vi "Update Tag String.vi"(8 "error in (no error)":errorcluster, 9 "string":string caption="String", 10 "Tag Path":string, 11 "Logger in.lvclass":refnum<class "Logger.lvclass">) -> (0 "error out":errorcluster, 3 "Logger out.lvclass":refnum<class "Logger.lvclass">)   [LabVIEW 2023, in "Logger.lvclass"]
uses:
  Logger.lvclass
  Logger.lvclass/Logger.ctl
  <vilib>/Skyline/Tag/Wrapper/Wrapper_class/Generate Tag Cluster (String) 2.vi
  <vilib>/Skyline/Tag/Wrapper/Wrapper_class/Generate Tag Cluster Core 2.vi
  <vilib>/Skyline/Tag/Wrapper/Wrapper_class/NI Skyline Tag.lvclass
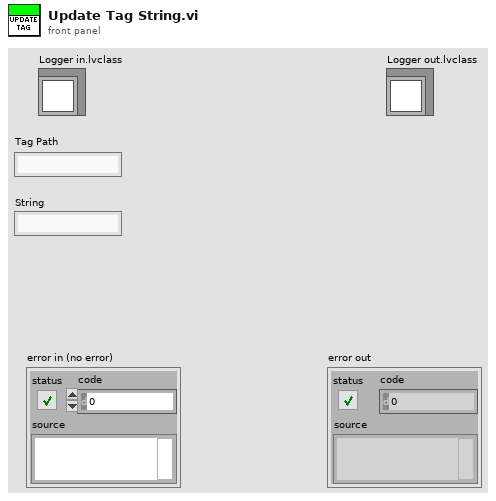
[diagram p1: front panel]
types:
  T1 = cluster{"Tag Units":string, "Tag Path":string, "Tag Reference":refnum<class "NI Skyline Tag.lvclass">}[]
  T2 = typedef "NI Skyline Tag.lvclass/Tag Value Cluster Wrapper.ctl" = cluster{"Configuration":refnum<class "NI Skyline Configuration.lvclass">, "Tag Cluster":T3}
  T3 = typedef "NI Skyline Tag.lvlib/Tag Value Cluster.ctl" = cluster{"Path":string, "Workspace ID":string, "Data Type":T4, "Value":string, "Time Stamp":timestamp}
  T4 = typedef "NI Skyline Tag.lvlib/DataType.ctl" = enum32{"Double", "I32", "String", "Boolean", "U64", "Timestamp"}
  T5 = cluster{"Tag Units":string, "Tag Path":string, "Tag Reference":refnum<class "NI Skyline Tag.lvclass">}
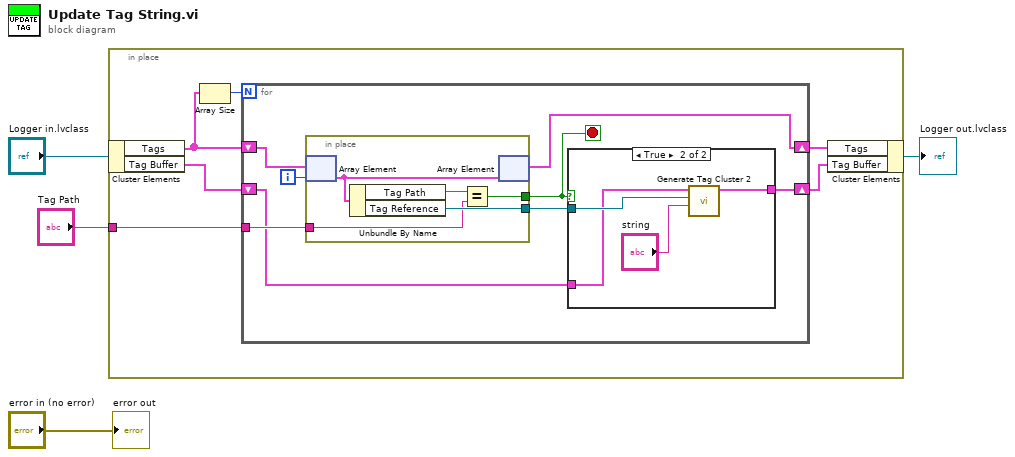
[diagram p0: block diagram]
diagram:
  n1 = in-place {
    in-place-border: "Tag Path" -> [w10]
    n2 = in-place-cluster #1("Logger in.lvclass") -> ("Tags"=w7:T1, "Tag Buffer"=w6:T2[])
    n3 = Array Size(array=w7) -> (size(s)=w8:i32)
    n4 = for {
      N: w8 -> [_]
      tunnel: w10 -> [w18]
      shift-right: [w13] -> w9
      shift-left: w7 -> [w17]
      shift-right: [w11] -> w5
      shift-left: w6 -> [w12]
      i -> [w16]
      stop <- w15 stop-if-true
      n5 = in-place {
        in-place-border: w18 -> [w24]
        in-place-border: [w26] -> w15
        in-place-border: [w28] -> w14
        n6 = in-place-array #2(w17, w16) -> (w27:T5)
        n7 = Unbundle By Name(w27) -> ("Tag Path"=w25:string, "Tag Reference"=w28:refnum<class "NI Skyline Tag.lvclass">)
        n8 = Equal?(x=w25, y=w24) -> (x = y?=w26:bool)
        n9 = in-place-array #2(w27) -> (w13:T1)  [unwired: 1 out]
      }
      n10 = case shown="True" w15 {
        tunnel: w14 -> [_ w23]
        tunnel: w12 -> [w19 w22]
        tunnel: [w19 w21] -> w11
        frame False {
        }
        frame True {
          n11 = call-poly <vilib>:"Generate Tag Cluster 2.vi"("value"="string", "tag in"=w23, "tag clusters in"=w22) -> ("tag clusters out"=w21:T2[])  [unwired: 6 in, 2 out]
        }
      }
    }
    n12 = in-place-cluster #1("Tags"=w9, "Tag Buffer"=w5) -> (→"Logger out.lvclass":refnum<class "Logger.lvclass">)
  }
  "error out" <- "error in (no error)"
